vi "Get Voltage RGB.vi"(3 "error in (no error)":errorcluster, 4 "Voltage":dbl) -> (0 "error out":errorcluster, 1 "RGB Value":u32)   [LabVIEW 2019]
doc: "This VI gets a color value (RGB) from a voltage."
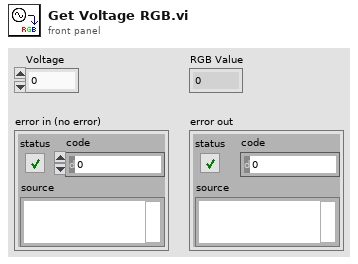
[diagram p1: front panel]
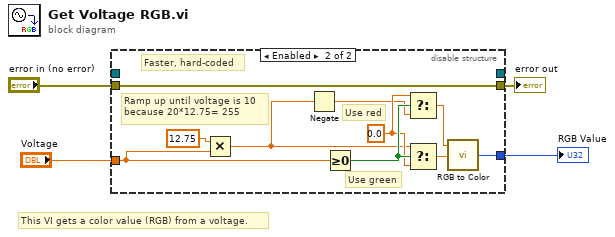
[diagram p0: block diagram]
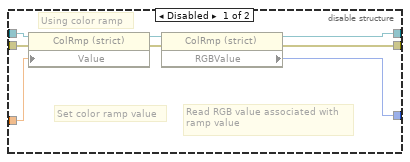
[diagram p2: hidden frame]
diagram:
  # "This VI gets a color value (RGB) from a voltage."
  n1 = disable-structure shown="Enabled" {
    disable-tunnel: [w12 w22] -> w1
    disable-tunnel: "Voltage" -> [w10 w19]
    disable-tunnel: "error in (no error)" -> [w8 w21]
    disable-tunnel: _ -> [w7 _]
    disable-tunnel: [w6 _] -> _
    disable-tunnel: [w5 w21] -> w2
    frame Disabled {
      # "Read RGB value associated with\nramp value"
      # "Set color ramp value"
      # "Using color ramp"
      n2 = property class="ColRmp (strict)"(reference=w7, error in=w8, "Value"=w10) -> (reference out=w9:refnum<vi>, error out=w11:errorcluster)
      n3 = property class="ColRmp (strict)"(reference=w9, error in=w11) -> (reference out=w6:refnum<vi>, error out=w5:errorcluster, "RGBValue"=w12:u32)
    }
    frame Enabled {
      w15 = 0.0 ("f")
      # "Use red"
      # "Use green"
      # "Ramp up until voltage is 10\nbecause 20*12.75= 255"
      # "Faster, hard-coded"
      n4 = Multiply(x=12.75, y=w19) -> (x*y=w14:dbl)
      n5 = Negate(x=w14) -> (-x=w13:dbl)
      n6 = Greater Or Equal To 0?(x=w19) -> (x >= 0?=w17:bool)
      n7 = Select(t=w15, s=w17, f=w13) -> (s? t:f=w16:dbl)
      n8 = Select(t=w14, s=w17, f=w15) -> (s? t:f=w18:dbl)
      n9 = call <vilib>:"RGB to Color.vi"("G"=w18, "R"=w16) -> ("Color"=w22:u32)  [unwired: 1 in]
    }
  }
  "RGB Value" <- w1
  "error out" <- w2
